vi "Get_detection_JSON.vi"() -> ()   [LabVIEW 2024]
panel:
  out "detection data":T1
  in  "index\n detections":i32
  out "detection":T2(array[cluster])
  out "annotated_image":string
  in  "path":path
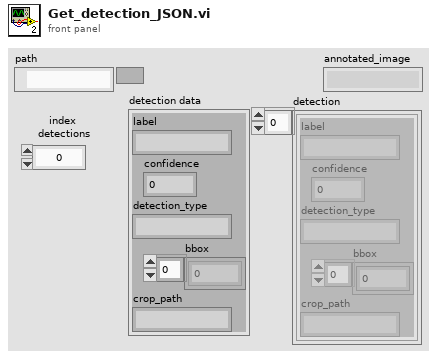
[diagram p1: front panel]
types:
  T1 = cluster{"label":string, "confidence":i32, "detection_type":string, "bbox":dbl[], "crop_path":string}
  T2 = cluster{"label":string, "confidence":i32, "detection_type":string, "bbox":dbl[], "crop_path":string}[]
  T3 = cluster{"annotated_image":string, "detections":cluster{"label":string, "confidence":i32, "detection_type":string, "bbox":dbl[], "crop_path":string}[]}
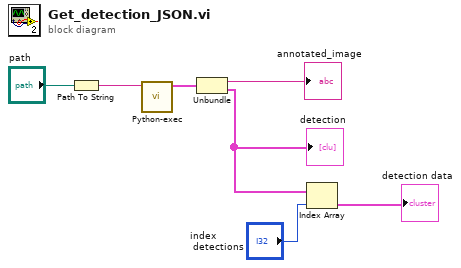
[diagram p0: block diagram]
diagram:
  n1 = Path To String(path="path") -> (string=w6:string)
  n2 = call "Python-exec.vi"("String"=w6) -> ("value"=w5:T3)  [unwired: 10 in]
  n3 = Unbundle(w5) -> ("annotated_image"=→"annotated_image":string, "detections"=w3:T2)
  "detection" <- w3
  n4 = Index Array(array=w3, index="index\n detections") -> (element=→"detection data":T1)
